vi "Columns.vi"() -> (2 "Columns":T1)   [LabVIEW 2020, in "Conditum-Example.lvlib" / "Game.lvclass"]
uses:
  Game.lvclass
  Columns.ctl
  Conditum/Columns/Entity/Entity.lvclass
  C:/dev/lv20CE/lv-conditum/Conditum/Columns/Relation/Relation.lvclass
  Conditum/Columns/Entity Collection/Entity Collection.lvclass
  Conditum/Columns/String/String.lvclass
  Conditum/Columns/Timestamp/Timestamp.lvclass
  Conditum/Columns/Boolean/Boolean.lvclass
  Conditum/Columns/Type/Definition.ctl
  Conditum/Relation Mapping.ctl
  Conditum/Columns/String/String Definition.ctl
  Conditum/Attributes.ctl
  Conditum/Columns/String/Definition.ctl
  User/User.lvclass
  Conditum/Columns/Timestamp/Timestamp Definition.ctl
  Conditum/Columns/Timestamp/Definition.ctl
  Conditum/Columns/Boolean/Boolean Definition.ctl
  Conditum/Columns/Boolean/Definition.ctl
  Conditum/Columns/Type/Type.lvclass/Type.ctl
  Conditum/Columns/Relation/Relation.lvclass/Relation.ctl
  Conditum/Columns/Relation/Define Relation.vi
  Conditum/Columns/Type/Define Type.vi
  Conditum/Columns/Relation/Relation.lvclass
  C:/dev/lv20CE/lv-conditum/Conditum/Columns/Type/Type.lvclass
  Game.lvclass/Game.ctl
  Conditum/Conditum.lvlib
  Conditum/Columns/Type/Type.lvclass
  Conditum/Entity/Entity.lvclass
  Conditum/Columns/Relation/Definition.ctl
  Conditum/Columns/Relation/Entity Relation Definition.ctl
  C:/dev/lv20CE/lv-conditum/Conditum/Entity/Entity.lvclass
  C:/dev/lv20CE/lv-conditum/Conditum-Example/User/User.lvclass
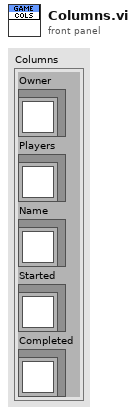
[diagram p1: front panel]
types:
  T1 = typedef "Conditum-Example.lvlib/Game.lvclass/Columns.ctl" = cluster{"Owner":refnum<class "Entity.lvclass">, "Players":refnum<class "Entity Collection.lvclass">, "Name":refnum<class "String.lvclass">, "Started":refnum<class "Timestamp.lvclass">, "Completed":refnum<class "Boolean.lvclass">}
  T2 = typedef "Conditum.lvlib/Columns.lvlib/Relation.lvclass/Entity Relation Definition.ctl" = cluster{"Type":T3, "Entity":T4}
  T3 = typedef "Conditum.lvlib/Columns.lvlib/Type.lvclass/Definition.ctl" = cluster{"Name":string, "Nullable":bool, "Default NULL":bool}
  T4 = typedef "Conditum.lvlib/Columns.lvlib/Relation.lvclass/Definition.ctl" = cluster{"Reversed By":string, "Mapping":T5, "Entity":refnum<class "Entity.lvclass">}
  T5 = typedef "Conditum.lvlib/Relation Mapping.ctl" = enum16{"OneToMany", "ManyToOne", "ManyToMany", "OneToOne"}
  T6 = typedef "Conditum.lvlib/Columns.lvlib/Boolean.lvclass/Boolean Definition.ctl" = cluster{"Type":T3, "Attributes":T7, "Boolean":T8}
  T7 = typedef "Conditum.lvlib/Attributes.ctl" = cluster{"Primary Key":bool, "Unique":bool, "Foreign Key":bool, "Auto Increment":bool}
  T8 = typedef "Conditum.lvlib/Columns.lvlib/Boolean.lvclass/Definition.ctl" = cluster{"Default":bool}
  T9 = typedef "Conditum.lvlib/Columns.lvlib/Timestamp.lvclass/Timestamp Definition.ctl" = cluster{"Type":T3, "Attributes":T7, "Timestamp":T10}
  T10 = typedef "Conditum.lvlib/Columns.lvlib/Timestamp.lvclass/Definition.ctl" = cluster{"Default":timestamp}
  T11 = typedef "Conditum.lvlib/Columns.lvlib/String.lvclass/String Definition.ctl" = cluster{"Type":T3, "Attributes":T7, "String":T12}
  T12 = typedef "Conditum.lvlib/Columns.lvlib/String.lvclass/Definition.ctl" = cluster{"Default":string, "Length":i32}
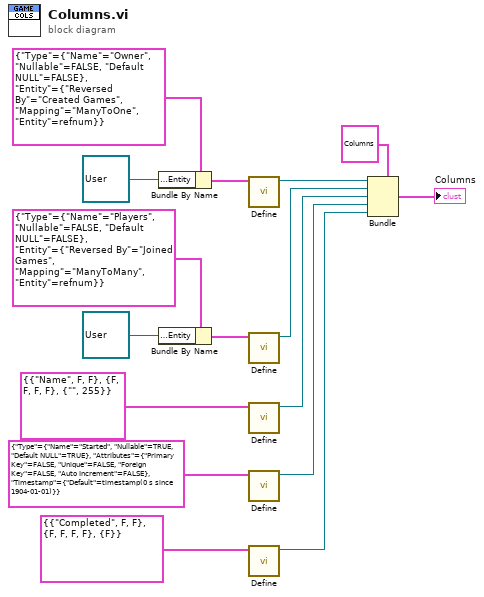
[diagram p0: block diagram]
diagram:
  n1 = Bundle By Name(cluster=T2 {"Type"={"Name"="Owner", "Nullable"=FALSE, "Default NULL"=FALSE}, "Entity"={"Reversed By"="Created Games", "Mapping"=enum."ManyToOne", "Entity"=refnum}} ("Entity Relation Definition"), "Entity.Entity"=refnum<class "User.lvclass"> refnum ("Conditum-Example.lvlib:User.lvclass")) -> (w1:T2)
  n2 = Bundle By Name(cluster=T2 {"Type"={"Name"="Players", "Nullable"=FALSE, "Default NULL"=FALSE}, "Entity"={"Reversed By"="Joined Games", "Mapping"=enum."ManyToMany", "Entity"=refnum}} ("Entity Relation Definition"), "Entity.Entity"=refnum<class "User.lvclass"> refnum ("Conditum-Example.lvlib:User.lvclass")) -> (w4:T2)
  n3 = call "Define.vi"("Entity Relation Definition"=w1) -> ("Entity out"=w13:refnum<class "Entity.lvclass">)  [unwired: 10 in]
  n4 = call "Define.vi"("Entity Relation Definition"=w4) -> ("Entity Collection out"=w12:refnum<class "Entity Collection.lvclass">)  [unwired: 10 in]
  n5 = call "Define.vi"("Definition"=T11 {"Type"={"Name"="Name", "Nullable"=FALSE, "Default NULL"=FALSE}, "Attributes"={"Primary Key"=FALSE, "Unique"=FALSE, "Foreign Key"=FALSE, "Auto Increment"=FALSE}, "String"={"Default"="", "Length"=255}}) -> ("String out"=w11:refnum<class "String.lvclass">)  [unwired: 10 in]
  n6 = call "Define.vi"("Definition"=T9 {"Type"={"Name"="Started", "Nullable"=TRUE, "Default NULL"=TRUE}, "Attributes"={"Primary Key"=FALSE, "Unique"=FALSE, "Foreign Key"=FALSE, "Auto Increment"=FALSE}, "Timestamp"={"Default"=timestamp(0 s since 1904-01-01)}}) -> ("DateTime out"=w10:refnum<class "Timestamp.lvclass">)  [unwired: 10 in]
  n7 = call "Define.vi"("Init Data"=T6 {"Type"={"Name"="Completed", "Nullable"=FALSE, "Default NULL"=FALSE}, "Attributes"={"Primary Key"=FALSE, "Unique"=FALSE, "Foreign Key"=FALSE, "Auto Increment"=FALSE}, "Boolean"={"Default"=FALSE}}) -> ("Boolean out"=w9:refnum<class "Boolean.lvclass">)  [unwired: 10 in]
  n8 = Bundle(cluster=T1 {"Owner"=refnum, "Players"=refnum, "Name"=refnum, "Started"=refnum, "Completed"=refnum} ("Columns"), "Owner"=w13, "Players"=w12, "Name"=w11, "Started"=w10, "Completed"=w9) -> (→"Columns":T1)
